vi "setUp.vi"(8 "error in (no error)":errorcluster, 11 "reference in":refnum<class "Test Numeric Test Object.lvclass">) -> (0 "error out":errorcluster, 3 "reference in":refnum<class "Test Numeric Test Object.lvclass">)   [LabVIEW 2009, in "Test Numeric Test Object.lvclass"]
doc: "setUp runs prior to the test method during test execution. Use this method to initialize any object data required by your tests."
uses:
  Test Numeric Test Object.lvclass
  Test Numeric Test Object.lvclass/Test Numeric Test Object.ctl
  <vilib>/addons/_JKI Toolkits/VI Tester/TestCase.llb/TestCase.lvclass
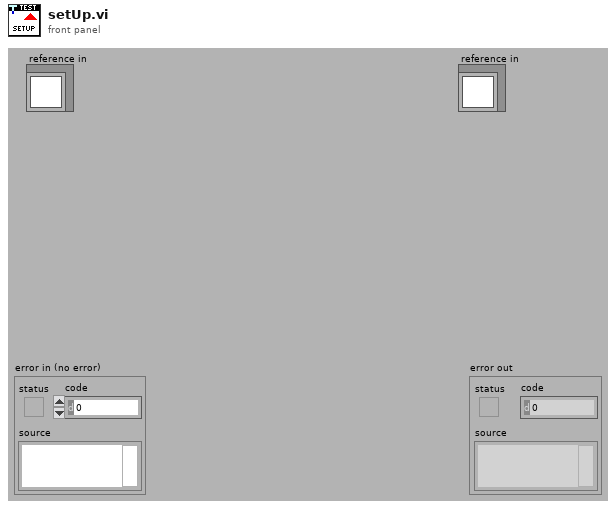
[diagram p1: front panel]
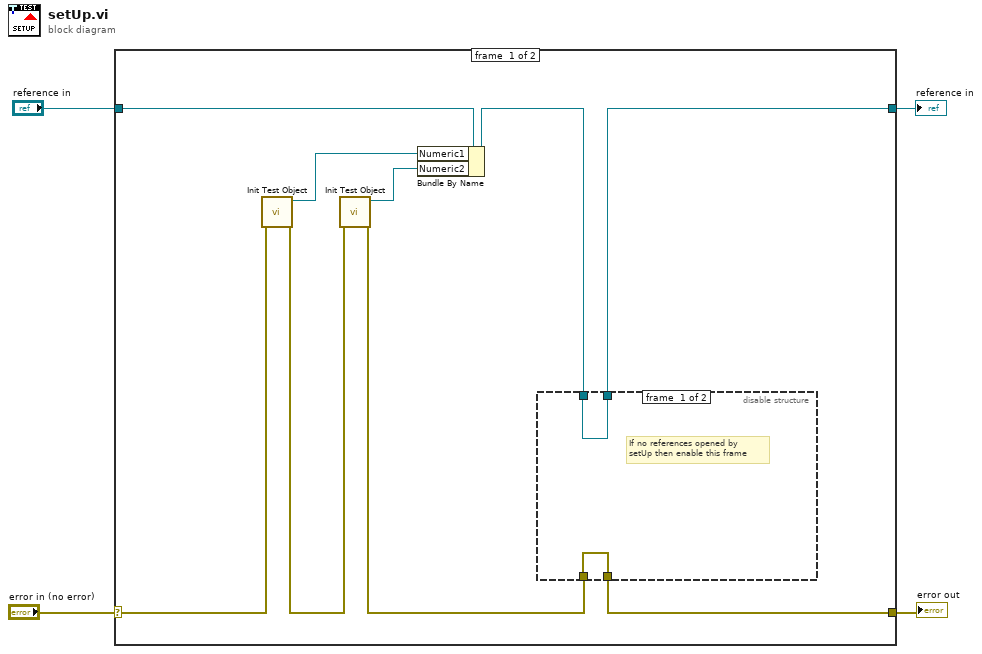
[diagram p0: block diagram]
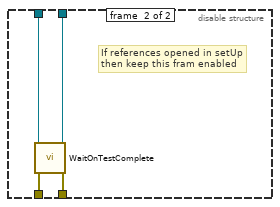
[diagram p2: hidden frame]
diagram:
  n1 = case shown="No Error" "error in (no error)" {
    selector: "error in (no error)" -> [w8 w21]
    tunnel: [w10 w21] -> w3
    tunnel: [w11 w20] -> w1
    tunnel: "reference in" -> [w13 w20]
    frame #0 {
      n2 = call "Init Test Object.vi"("error in (no error)"=w8) -> ("error out"=w7:errorcluster, "Numeric out"=w9:refnum<class "Numeric Test Object.lvclass">)  [unwired: 9 in]
      n3 = call "Init Test Object.vi"("error in (no error)"=w7) -> ("error out"=w6:errorcluster, "Numeric out"=w5:refnum<class "Numeric Test Object.lvclass">)  [unwired: 9 in]
      n4 = Bundle By Name(cluster=w13, "Numeric1"=w9, "Numeric2"=w5) -> (w12:refnum<class "Test Numeric Test Object.lvclass">)
      n5 = disable-structure shown="Enabled" {
        disable-tunnel: w12 -> [w15 w19]
        disable-tunnel: [w15 w18] -> w11
        disable-tunnel: w6 -> [w14 w17]
        disable-tunnel: [w14 w16] -> w10
        frame #0 {
          # "If no references opened by\nsetUp then enable this frame"
        }
        frame #1 {
          # "If references opened in setUp\nthen keep this fram enabled"
          n6 = call <vilib>:"WaitOnTestComplete.vi"("error in (no error)"=w17, "TestCase in"=w19) -> ("error out"=w16:errorcluster, "TestCase out"=w18:refnum<class "Test Numeric Test Object.lvclass">)  [unwired: 8 in]
        }
      }
    }
    frame #1 {
    }
  }
  "error out" <- w3
  "reference in" <- w1
